vi "Cmd to R_W - Asynchronous.vi"(8 "error in":errorcluster, 9 "Write Only?":bool, 10 "write buffer":string, 11 "Serial IO in":refnum<class "Serial IO.lvclass">) -> (0 "error out":errorcluster, 2 "read buffer":string, 3 "Serial IO out":refnum<class "Serial IO.lvclass">)   [LabVIEW 2015, in "Serial IO.lvclass"]
doc: "In most instances, retrieval of data from a serial port is commenced with a write. This VI writes to the port and then waits for a response. Depending on the configuration, the VISA read will be based on:\n1) A specified amount of time for bytes to become available before perfomring a read on that port. These parameters (as well as the port enumeration) are located in the superclass.\n2) For the end as defined by the parameter ASRL End In.\nIf (2) is not defined in the device configuration then the execution of this VI will proceed using the wait for bytes loop found in case 0.\n\n<B>This VI is reentrant to allow access to the different ports that different devices might be communicating with simultaneously.</B>"
uses:
  Serial IO.lvclass
  Serial IO.lvclass/Serial IO.ctl
  <vilib>/Platform/TimedLoop/XDataNode/timing_clust.ctl
  <vilib>/Platform/TimedLoop/XDataNode/nitl_modes.ctl
  <vilib>/Platform/TimedLoop/XDataNode/wakeup.ctl
  <vilib>/Platform/TimedLoop/XDataNode/XDataNode.xnode
  <vilib>/Platform/TimedLoop/XDataNode/XDNodeRunTimeDep.lvlib
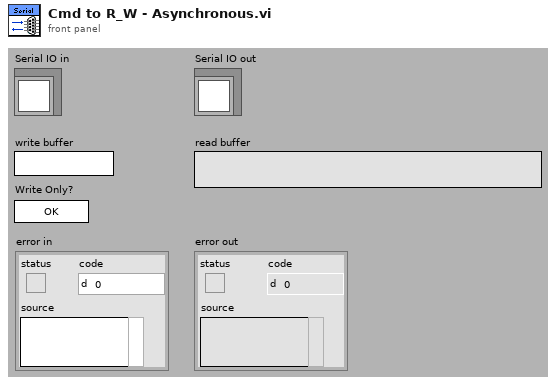
[diagram p1: front panel]
types:
  T1 = typedef "XDNodeRunTimeDep.lvlib/timing_clust.ctl" = cluster{"Expected End [f-1]":u64, "Actual End [f-1]":u64, "Finished Late? [f-1]":bool, "Expected End [i-1]":u64, "Actual End [i-1]":u64, "Finished Late? [i-1]":bool, "Expected Start [i]":u64, "Actual Start [i]":u64, "Expected Start [f]":u64, "Actual Start [f]":u64, "Source Name":string, "Structure Name":string, "Period":i64, "Deadline":i64, "Offset":i64, "Start":i64, "Priority":i32, "Timeout":i32, "Mode":T2, "Wakeup Reason":T3, "Error":errorcluster, "Source Type":string, "Secondary Source Type":string, "Global End Time":u64, "Global Start Time":u64, "Frame Duration":u64, "Iteration Duration":u64, "Assigned CPU":i32, "I/O Scan Engine Mode":u32}
  T2 = typedef "XDNodeRunTimeDep.lvlib/nitl_modes.ctl" = enum32{"No Change", "Process missed periods, maintain original phase", "Discard missed periods, maintain original phase", "Process missed periods, ignore original phase", "Discard missed periods, ignore original phase"}
  T3 = typedef "XDNodeRunTimeDep.lvlib/wakeup.ctl" = enum32{"Normal", "Aborted", "Asynchronous wakeup", "Timing source error", "Timed loop error", "Timeout"}
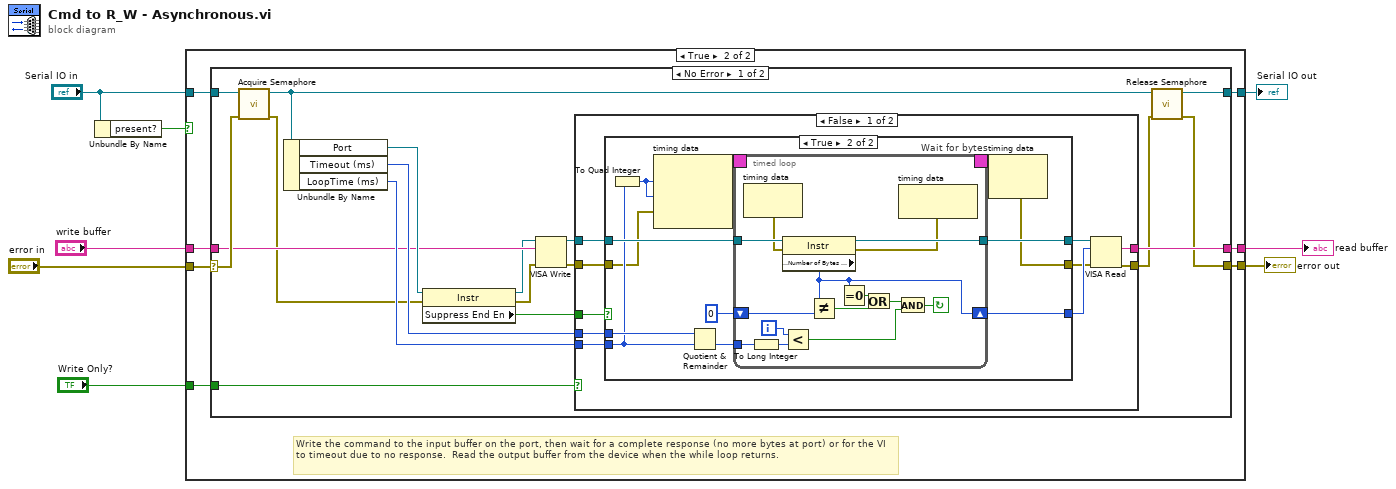
[diagram p0: block diagram]
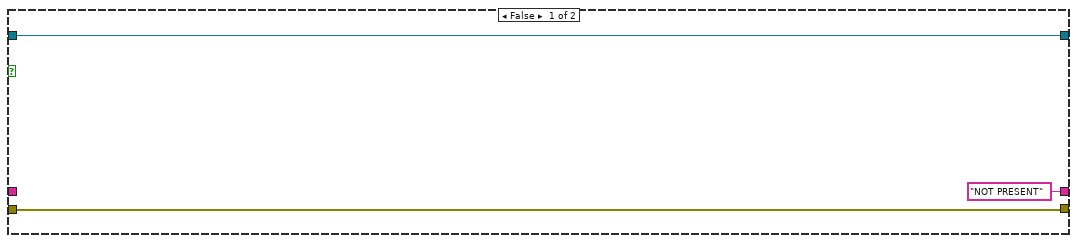
[diagram p2: hidden frame]
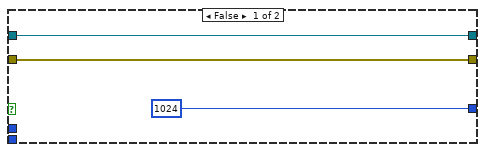
[diagram p3: hidden frame]
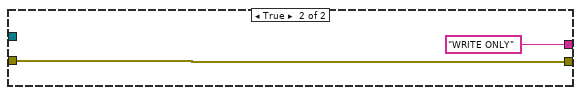
[diagram p4: hidden frame]
diagram:
  n1 = Unbundle By Name("Serial IO in") -> ("present?"=w1:bool)
  n2 = case shown="True" w1 {
    tunnel: [w11 w18] -> w8
    tunnel: "Serial IO in" -> [w11 w17]
    tunnel: "error in" -> [w9 w16]
    tunnel: [w9 w15] -> w6
    tunnel: ["NOT PRESENT" ("read buffer") w14] -> w5
    tunnel: "write buffer" -> [_ w13]
    tunnel: "Write Only?" -> [_ w12]
    frame False {
    }
    frame True {
      # "Write the command to the input buffer on the port, then wait for a complete response (no more bytes at port) or for the VI to timeout due to no response.  Read the output buffer from the device when the while loop returns."
      n3 = case shown="No Error" w16 {
        selector: w16 -> [w28 w91]
        tunnel: [w24 w91] -> w15
        tunnel: [w26 w90] -> w18
        tunnel: [w32 _] -> w14
        tunnel: w17 -> [w29 w90]
        tunnel: w13 -> [w23 _]
        tunnel: w12 -> [w19 _]
        frame No Error {
          n4 = call "Acquire Semaphore.vi"("error in"=w28, "Serial IO in"=w29) -> ("error out"=w22:errorcluster, "Serial IO out"=w27:refnum<class "Serial IO.lvclass">)  [unwired: 8 in]
          n5 = Unbundle By Name(w27) -> ("Port"=w31:refnum<visa-resource-name>, "Timeout (ms)"=w35:u32, "LoopTime (ms)"=w34:u32)
          n6 = property class="Instr"(reference=w31, error in=w22) -> (reference out=w21:refnum<visa-resource-name>, error out=w20:errorcluster, "Suppress End En"=w30:bool)
          n7 = VISA Write(VISA resource name=w21, write buffer=w23, error in (no error)=w20) -> (VISA resource name out=w36:refnum<visa-resource-name>, error out=w33:errorcluster)  [unwired: 1 out]
          n8 = case shown="False" w19 {
            tunnel: w36 -> [w46 _]
            tunnel: w35 -> [w43 _]
            tunnel: w34 -> [w42 _]
            tunnel: w33 -> [w41 w89]
            tunnel: [w39 "WRITE ONLY" ("read buffer")] -> w32
            tunnel: w30 -> [w38 _]
            tunnel: [w37 w89] -> w25
            frame False {
              n9 = case shown="True" w38 {
                tunnel: w46 -> [w48 w59]
                tunnel: [w48 w58] -> w45
                tunnel: [u32 1024 w57] -> w44
                tunnel: w43 -> [_ w56]
                tunnel: w42 -> [_ w55]
                tunnel: w41 -> [w49 w54]
                tunnel: [w49 w53] -> w40
                frame False {
                }
                frame True {
                  n10 = To Quad Integer(1:w55) -> (0:w50:i64)
                  n11 = node-c288(w50, w50, w54) -> (w61:T1)
                  n12 = Quotient & Remainder(x=w56, y=w55) -> (floor(x/y)=w52:u32)  [unwired: 1 out]
                  n13 = timed-loop "Wait for bytes" {
                    tunnel: w59 -> [w75]
                    tunnel: [w74] -> w58
                    tunnel: w52 -> [w63]
                    shift-right: [w66] -> w57
                    shift-left: u32 0 -> [w67]
                    timing: w61 -> [_]
                    timing-out: [_] -> w60
                    i -> [w73]
                    stop <- w72 continue-if-true
                    n14 = node-c288() -> (w65:errorcluster)  [unwired: 1 in]
                    n15 = To Long Integer(number=w63) -> (32bit integer=w62:i32)
                    n16 = property class="Instr"(reference=w75, error in=w65) -> (reference out=w74:refnum<visa-resource-name>, error out=w64:errorcluster, "Serial Settings:Number of Bytes at Serial Port"=w66:u32)
                    n17 = Less?(x=w73, y=w62) -> (x < y?=w71:bool)
                    n18 = Not Equal?(x=w66, y=w67) -> (x != y?=w70:bool)
                    n19 = Equal To 0?(x=w66) -> (x = 0?=w69:bool)
                    n20 = Or(x=w69, y=w70) -> (x .or. y?=w68:bool)
                    n21 = And(x=w68, y=w71) -> (x .and. y?=w72:bool)
                    n22 = node-c288(w64) -> ()  [unwired: 1 out]
                  }
                  n23 = node-c288(w60) -> (w53:errorcluster)
                }
              }
              n24 = VISA Read(VISA resource name=w45, byte count=w44, error in (no error)=w40) -> (read buffer=w39:string, error out=w37:errorcluster)  [unwired: 2 out]
            }
            frame True {
            }
          }
          n25 = call "Release Semaphore.vi"("error in (no error)"=w25, "Serial IO in"=w27) -> ("error out"=w24:errorcluster, "Serial IO out"=w26:refnum<class "Serial IO.lvclass">)  [unwired: 8 in]
        }
        frame Error {
        }
      }
    }
  }
  "Serial IO out" <- w8
  "error out" <- w6
  "read buffer" <- w5
